vi "Ustaw widocznosc kontrolek.vi"(7 "Disabled/Enabled":T2(ring), 9 "Klaster referencji":T1) -> ()   [LabVIEW 2015]
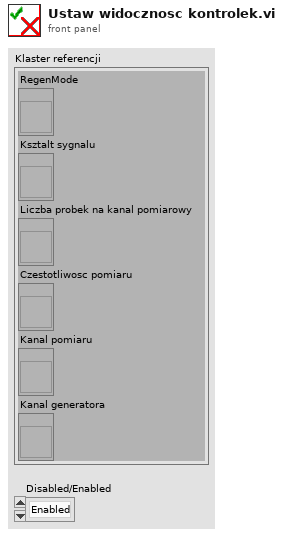
[diagram p1: front panel]
types:
  T1 = cluster{"RegenMode":refnum<vi>, "Ksztalt sygnalu":refnum<vi>, "Liczba probek na kanal pomiarowy":refnum<vi>, "Czestotliwosc pomiaru":refnum<vi>, "Kanal pomiaru":refnum<vi>, "Kanal generatora":refnum<vi>}
  T2 = enum8{"Enabled", "Disabled", "Disabled and Grayed Out"}
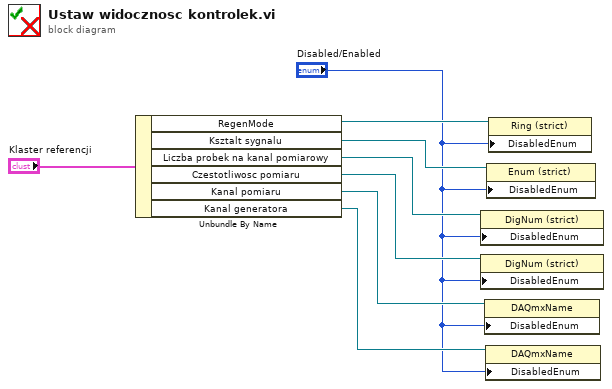
[diagram p0: block diagram]
diagram:
  n1 = Unbundle By Name("Klaster referencji") -> ("RegenMode"=w8:refnum<vi>, "Ksztalt sygnalu"=w6:refnum<vi>, "Liczba probek na kanal pomiarowy"=w5:refnum<vi>, "Czestotliwosc pomiaru"=w4:refnum<vi>, "Kanal pomiaru"=w3:refnum<vi>, "Kanal generatora"=w2:refnum<vi>)
  n2 = property class="DigNum (strict)"(reference=w5, "DisabledEnum"="Disabled/Enabled") -> ()  [unwired: 1 in, 2 out]
  n3 = property class="DigNum (strict)"(reference=w4, "DisabledEnum"="Disabled/Enabled") -> ()  [unwired: 1 in, 2 out]
  n4 = property class="DAQmxName"(reference=w3, "DisabledEnum"="Disabled/Enabled") -> ()  [unwired: 1 in, 2 out]
  n5 = property class="DAQmxName"(reference=w2, "DisabledEnum"="Disabled/Enabled") -> ()  [unwired: 1 in, 2 out]
  n6 = property class="Enum (strict)"(reference=w6, "DisabledEnum"="Disabled/Enabled") -> ()  [unwired: 1 in, 2 out]
  n7 = property class="Ring (strict)"(reference=w8, "DisabledEnum"="Disabled/Enabled") -> ()  [unwired: 1 in, 2 out]
